vi "_Convert Virtual Channel.vi"(2 "DAC":u32, 3 "Ch#":u8) -> (0 "DAC Out":u32, 1 "Ch# Out":u8)   [LabVIEW 2012]
uses:
  Type/_FPGA Chip Type.ctl
  <vilib>/rvi/eio/common/nirviEmuTemplateMethod_errors.vi
  <vilib>/eio/EIONode/EIONode.xnode
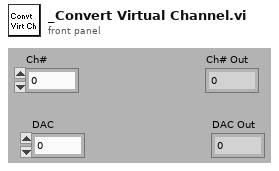
[diagram p1: front panel]
types:
  T1 = typedef "_FPGA Chip Type.ctl" = enum8{"None", "ADC1", "ADC2", "ADC3", "ADC4", "ADC5", "ADC6", "ADC7", "ADC8", "ADC9", "ADC10", "ADC11", "ADC12", "ADC13", "DAC1", "DAC2", "DAC3", "DAC4", "DAC5", "LENS1", "LENS2", "LENS3", "LENS4", "LENS5", "LENS6", "LENS7", "MASS1", "MASS2", "MASS3", "MASS4", "MASS5", "OSC1", "OSC2", "OSC3", "LATCH1", "LATCH2", "LATCH3", "LATCH4", "PIC1", "PIC2", "PIC3", "PIC4"}
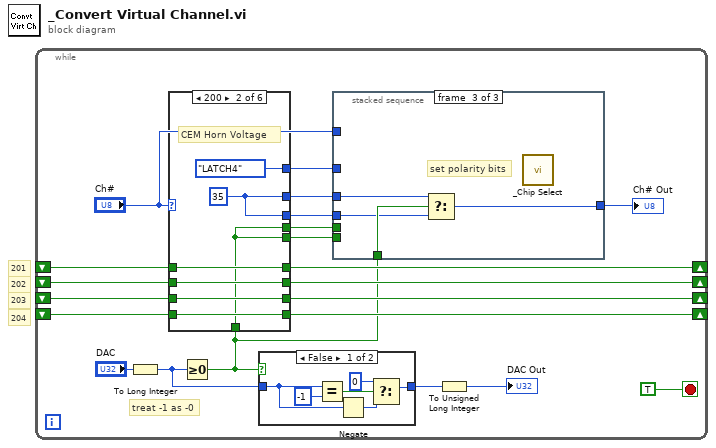
[diagram p0: block diagram]
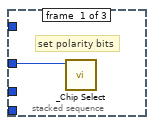
[diagram p3: hidden frame]
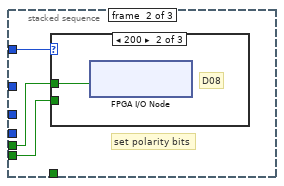
[diagram p4: hidden frame]
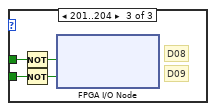
[diagram p6: hidden frame]
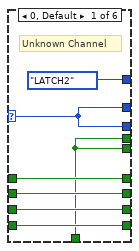
[diagram p7: hidden frame]
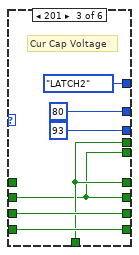
[diagram p8: hidden frame]
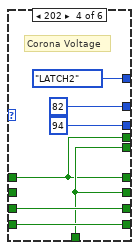
[diagram p9: hidden frame]
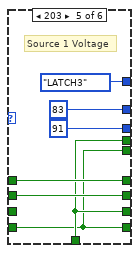
[diagram p10: hidden frame]
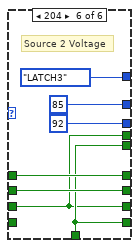
[diagram p11: hidden frame]
diagram:
  # "204"
  # "203"
  # "202"
  # "201"
  n1 = while {
    shift-right: [w16] -> _
    shift-left: _ -> [w12]
    shift-right: [w15] -> _
    shift-left: _ -> [w11]
    shift-right: [w14] -> _
    shift-left: _ -> [w10]
    shift-right: [w13] -> _
    shift-left: _ -> [w9]
    stop <- TRUE stop-if-true
    # "treat -1 as -0"
    n2 = To Long Integer(number="DAC") -> (32bit integer=w3:i32)
    n3 = Greater Or Equal To 0?(x=w3) -> (x >= 0?=w2:bool)
    n4 = case shown="200" "Ch#" {
      selector: "Ch#" -> [w48 _ _ _ _ _]
      tunnel: [w48 w54 u8 80 ("y") u8 82 ("y") u8 83 ("y") u8 85 ("y")] -> w7
      tunnel: [w48 w54 u8 93 ("y") u8 94 ("y") u8 91 ("y") u8 92 ("y")] -> w6
      tunnel: [_FPGA_Chip_Type."LATCH2" ("ChipType") _FPGA_Chip_Type."LATCH4" ("ChipType") _FPGA_Chip_Type."LATCH2" ("ChipType") _FPGA_Chip_Type."LATCH2" ("ChipType") _FPGA_Chip_Type."LATCH3" ("ChipType") _FPGA_Chip_Type."LATCH3" ("ChipType")] -> w8
      tunnel: w2 -> [w42 w49 w57 w64 w71 w78]
      tunnel: [w46 w50 w57 w63 w72 w79] -> w16
      tunnel: [w45 w53 w56 w64 w73 w80] -> w15
      tunnel: [w44 w52 w59 w66 w71 w77] -> w14
      tunnel: [w43 w51 w58 w65 w70 w78] -> w13
      tunnel: w11 -> [w45 w53 w56 _ w73 w80]
      tunnel: w10 -> [w44 w52 w59 w66 _ w77]
      tunnel: w9 -> [w43 w51 w58 w65 w70 _]
      tunnel: w12 -> [w46 w50 _ w63 w72 w79]
      tunnel: [w42 w49 w57 w63 w71 w77] -> w5
      tunnel: [w42 w49 w56 w64 w70 w78] -> w4
      frame 0, Default {
        # "Unknown Channel"
      }
      frame 200 {
        w54 = u8 35 ("y")
        # "CEM Horn Voltage"
      }
      frame 201 {
        # "Cur Cap Voltage"
      }
      frame 202 {
        # "Corona Voltage"
      }
      frame 203 {
        # "Source 1 Voltage"
      }
      frame 204 {
        # "Source 2 Voltage"
      }
    }
    n5 = case shown="False" w2 {
      tunnel: [w26 w28] -> w1
      tunnel: w3 -> [w23 w28]
      frame False {
        n6 = Equal?(x=w23, y=-1) -> (x = y?=w25:bool)
        n7 = Negate(x=w23) -> (-x=w22:i32)
        n8 = Select(t=0 ("y"), s=w25, f=w22) -> (s? t:f=w26:i32)
      }
      frame True {
      }
    }
    n9 = stacked-sequence {
      tunnel: w8 -> [w29 _ _]
      tunnel: w2 -> [_ _ w41]
      tunnel: "Ch#" -> [_ w32 _]
      tunnel: w7 -> [_ _ w40]
      tunnel: w6 -> [_ _ w39]
      tunnel: [_ _ w38] -> w20
      tunnel: w5 -> [_ w31 _]
      tunnel: w4 -> [_ w30 _]
      frame #0 {
        # "set polarity bits"
        n10 = call "_Chip Select.vi"("ChipType"=w29) -> ()  [unwired: 1 in, 6 out]
      }
      frame #1 {
        # "set polarity bits"
        n11 = case shown="200" w32 {
          tunnel: w31 -> [_ w33 w37]
          tunnel: w30 -> [_ _ w36]
          frame 0, Default {
          }
          frame 200 {
            # "D08"
            n12 = xnode "FPGA I/O Node"("Port4/DIO0"=w33) -> ()  [unwired: 1 in, 1 out]
          }
          frame 201..204 {
            # "D09"
            # "D08"
            n13 = Not(x=w37) -> (.not. x?=w35:bool)
            n14 = Not(x=w36) -> (.not. x?=w34:bool)
            n15 = xnode "FPGA I/O Node"("Port4/DIO0"=w35, "Port3/DIO8"=w34) -> ()  [unwired: 2 in, 2 out]
          }
        }
      }
      frame #2 {
        # "set polarity bits"
        n16 = Select(t=w40, s=w41, f=w39) -> (s? t:f=w38:u8)
        n17 = call "_Chip Select.vi"() -> ()  [unwired: 2 in, 6 out]
      }
    }
    "Ch# Out" <- w20
    n18 = To Unsigned Long Integer(number=w1) -> (unsigned 32bit integer=→"DAC Out":u32)
  }
